vi "BUFMGR_Release_Buffer.vi"(0 "Buffer Name":string, 5 "buffer in":u64, 11 "error in (no error)":errorcluster) -> (4 "return":u32 format="%.0x", 6 "released buffer":u64, 15 "error out":errorcluster)   [LabVIEW 2016]
uses:
  c/lib/libbuf.so
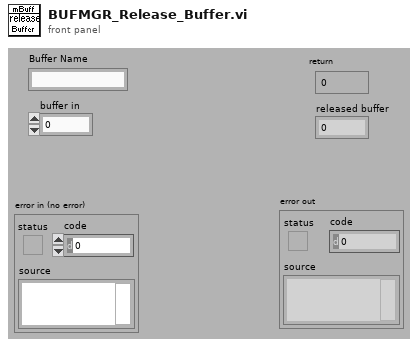
[diagram p1: front panel]
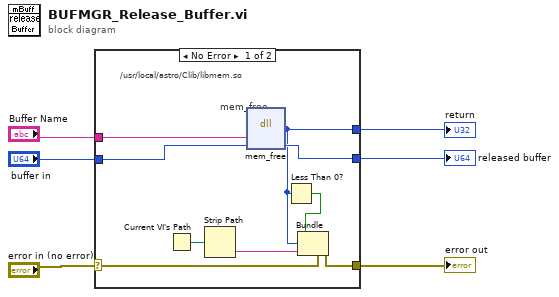
[diagram p0: block diagram]
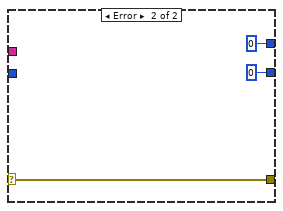
[diagram p2: hidden frame]
diagram:
  n1 = case shown="No Error" "error in (no error)" {
    selector: "error in (no error)" -> [w7 w16]
    tunnel: "Buffer Name" -> [w15 _]
    tunnel: [w10 u32 0] -> w5
    tunnel: "buffer in" -> [w14 _]
    tunnel: [w13 u64 0 ("size")] -> w3
    tunnel: [w12 w16] -> w2
    frame No Error {
      # "/usr/local/astro/Clib/libmem.so"
      # "mem_free"
      n2 = Current VI's Path() -> (path=w9:path)
      n3 = Strip Path(path=w9) -> (name=w8:string)  [unwired: 1 out]
      n4 = dll-call lib="home/simager/panview/PAN/Modules/buffermgr/private/c/lib/libbuf.so" fn="mem_free"("name"=w15, "buffer"=w14) -> ("return type"=w10:u32, "buffer"=w13:u64)  [unwired: 4 in, 2 out]
      n5 = Less Than 0?(x=w10) -> (x < 0?=w11:bool)
      n6 = Bundle(cluster=w7, "status"=w11, "code"=w10, "source"=w8) -> (w12:errorcluster)
    }
    frame Error {
    }
  }
  "error out" <- w2
  "return" <- w5
  "released buffer" <- w3
